vi "generateINIexclusionlist.vi"(11 "T for reso, F for galvo":bool) -> (3 "Array":string[](array[string]))   [LabVIEW 2012]
doc: "SciScan 1.2 160622"
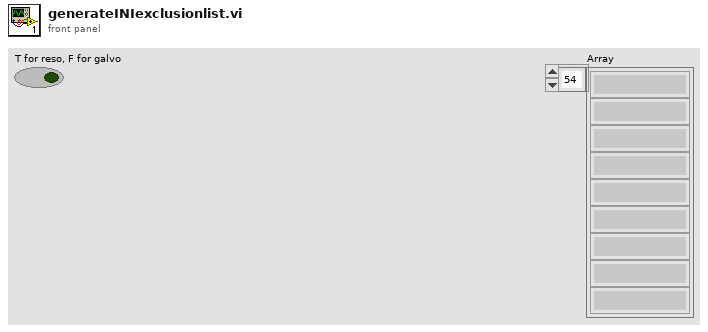
[diagram p1: front panel]
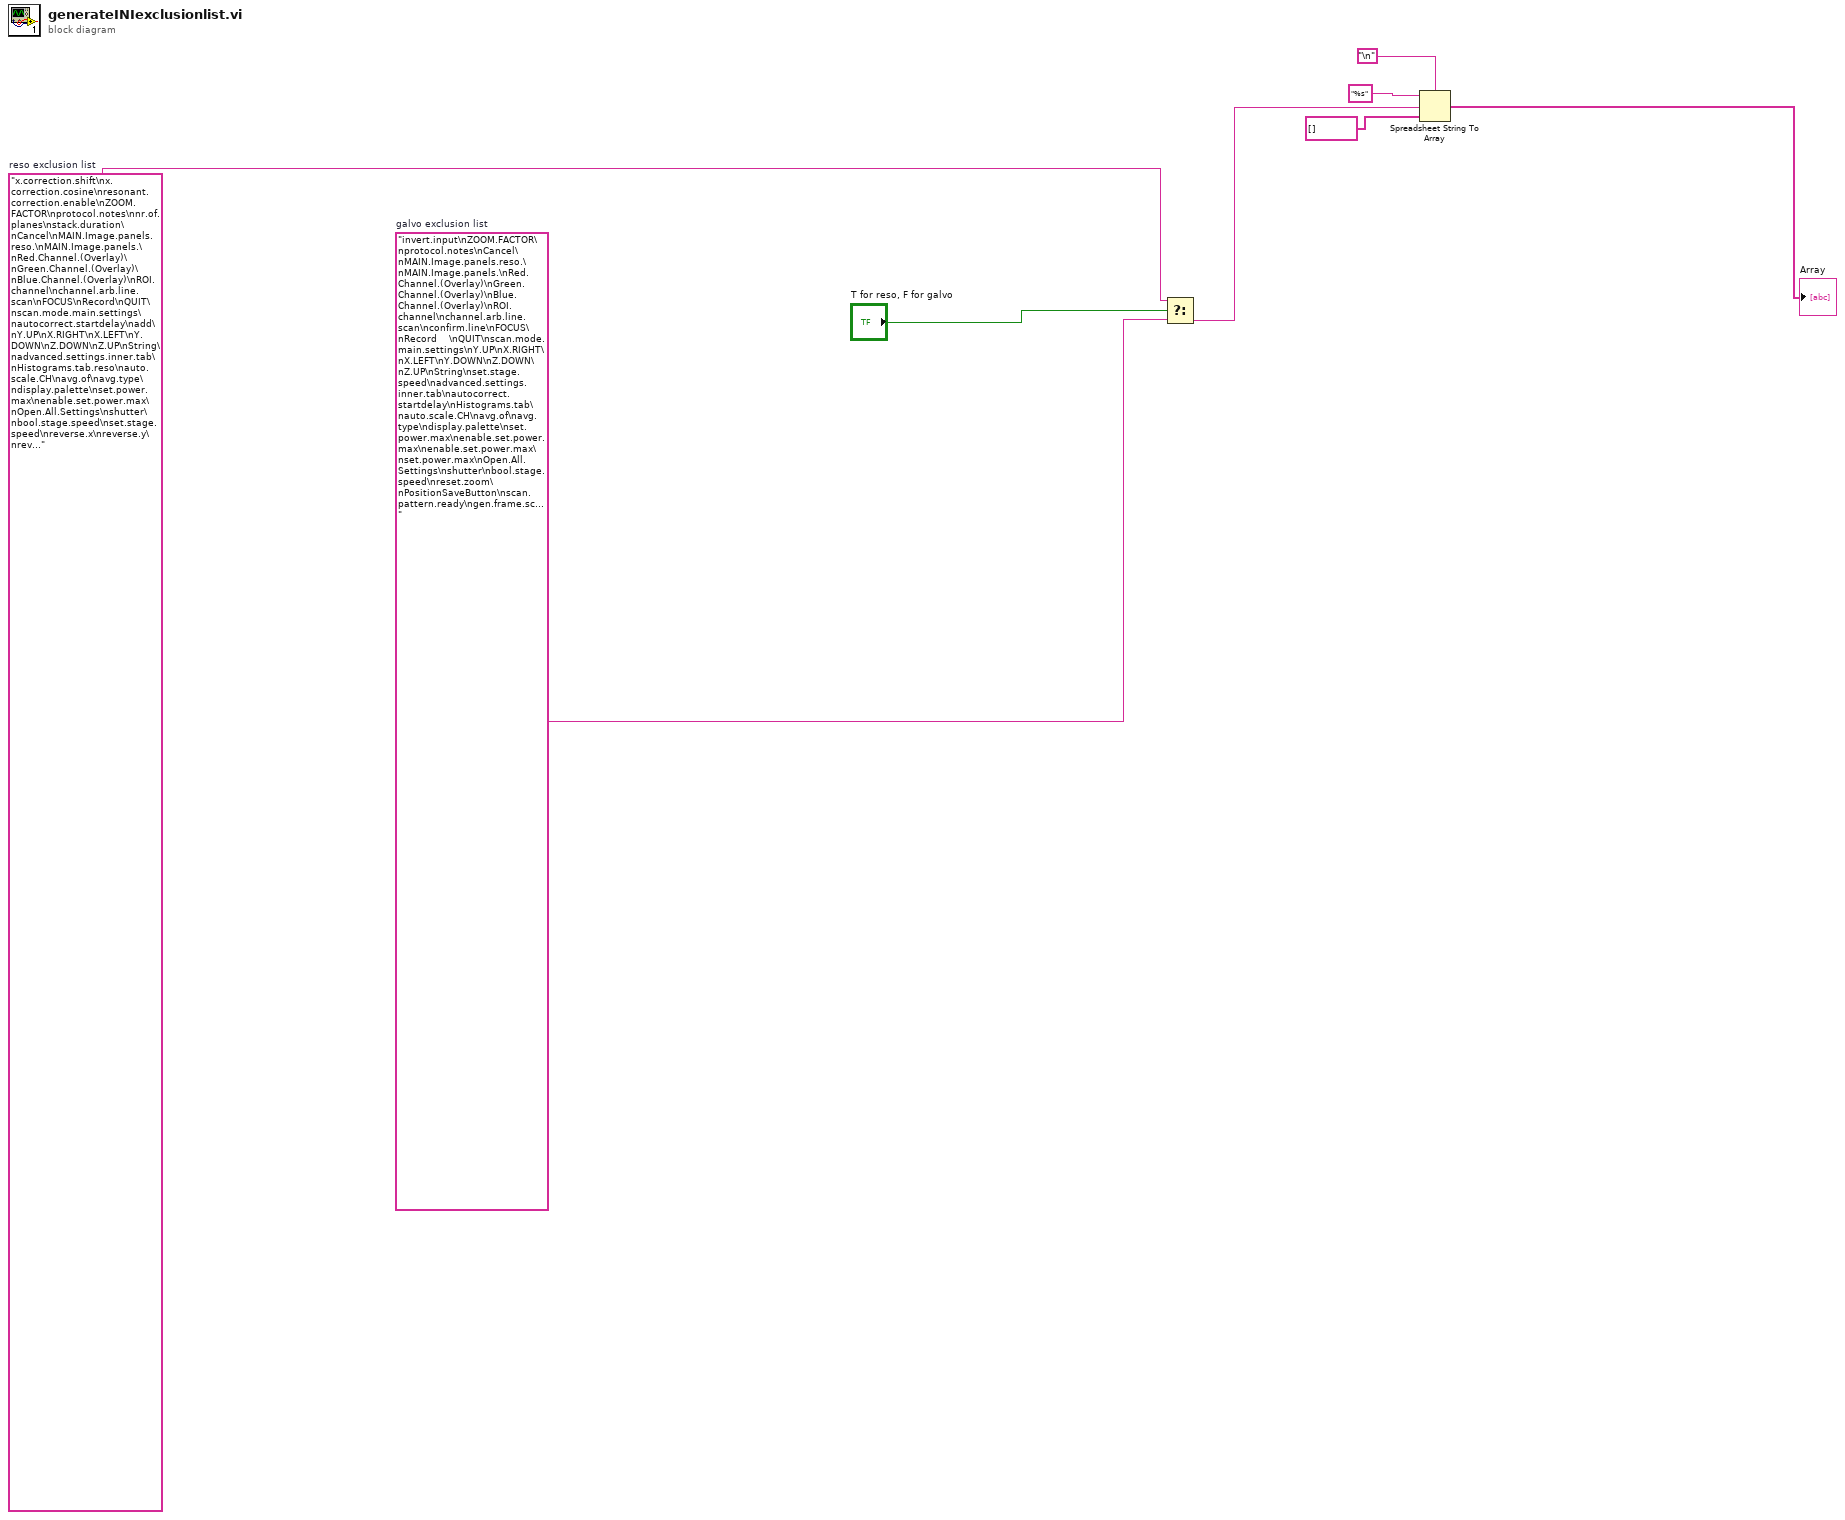
[diagram p0: block diagram]
diagram:
  w2 = "x.correction.shift\nx.correction.cosine\nresonant.correction.enable\nZOOM.FACTOR\nprotocol.notes\nnr.of.planes\nstack.duration\nCancel\nMAIN.Image.panels.reso.\nMAIN.Image.panels.\nRed.Channel.(Overlay)\nGreen.Channel.(Overlay)\nBlue.Channel.(Overlay)\nROI.channel\nchannel.arb.line.scan\nFOCUS\nRecord\nQUIT\nscan.mode.main.settings\nautocorrect.startdelay\nadd\nY.UP\nX.RIGHT\nX.LEFT\nY.DOWN\nZ.DOWN\nZ.UP\nString\nadvanced.settings.inner.tab\nHistograms.tab.reso\nauto.scale.CH\navg.of\navg.type\ndisplay.palette\nset.power.max\nenable.set.power.max\nOpen.All.Settings\nshutter\nbool.stage.speed\nset.stage.speed\nreverse.x\nreverse.y\nreverse.z\nLP.enable\nPositionSaveButton\nflystop\nposY.2\nposX.2\nposZ.2\nmodulesloaded\nsetZ.2\nsetX.2\nsetY.2\nX.RIGHT.2\nY.DOWN.2\nX.LEFT.2\nY.UP.2\nstep.size.xy.2\nZ.DOWN.2\nZ.UP.2\nstep.size.z.2\nSource\nOverlay\nHide\nauto.scale.Red.\nauto.scale.Green\nFOCUS2\nPSM.buttons.registered\nPreview.Mode\nSciScript_MD_first_launch\nflystart\nchannel.no\nScan_Complete\nno.of.frames.for.frame.scan\nSettings.Confirmed\nMacroExecTimeRemaining\nslider\ndisplay.every.n-th.frame\nObjective\nnomin.x.pixels\nrun.z.stack\nMICpos\nMICset\nObjective\nImageJ.path\npockels.maxpower\nframes.p.sec\nx.volt.offset\ny.volt.offset"  # reso exclusion list
  w8 = "invert.input\nZOOM.FACTOR\nprotocol.notes\nCancel\nMAIN.Image.panels.reso.\nMAIN.Image.panels.\nRed.Channel.(Overlay)\nGreen.Channel.(Overlay)\nBlue.Channel.(Overlay)\nROI.channel\nchannel.arb.line.scan\nconfirm.line\nFOCUS\nRecord    \nQUIT\nscan.mode.main.settings\nY.UP\nX.RIGHT\nX.LEFT\nY.DOWN\nZ.DOWN\nZ.UP\nString\nset.stage.speed\nadvanced.settings.inner.tab\nautocorrect.startdelay\nHistograms.tab\nauto.scale.CH\navg.of\navg.type\ndisplay.palette\nset.power.max\nenable.set.power.max\nenable.set.power.max\nset.power.max\nOpen.All.Settings\nshutter\nbool.stage.speed\nreset.zoom\nPositionSaveButton\nscan.pattern.ready\ngen.frame.scan\nrun.z.stack\nposY.2\nposX.2\nposZ.2\nsetX.2\nsetY.2\nsetZ.2\nstep.size.z\nSource\nOverlay\nHide\nauto.scale.Red\nauto.scale.Green\nFOCUS2\nPSM.buttons.registered\nmodulesloaded\nPreview.Mode\nflystop\nflystart\nchannel.no\nScan_Complete\nMacroExecTimeRemaining\nslider"  # galvo exclusion list
  n1 = Select(t=w2, s="T for reso, F for galvo", f=w8) -> (s? t:f=w3:string)
  n2 = Spreadsheet String To Array(delimiter (Tab)="\n", format string="%s", spreadsheet string=w3, array type (2D Dbl)=string[] []) -> (array=→"Array":string[])
